vi "Request Vecto Info.vi"(8 "error in (no error)":errorcluster, 9 "Timeout mS (1000)":i32=1000, 11 "VectoService in":refnum<class "VectoInfo.lvclass">) -> (0 "error out":errorcluster, 2 "Vecto Info":T1, 3 "VectoService out":refnum<class "VectoInfo.lvclass">)   [LabVIEW 2020, in "Vecto.lvlib" / "VectoInfo.lvclass"]
uses:
  VectoInfo.lvclass
  lv-promises/Promises/Future/Future.lvclass
  lv-promises/Promises/Promise/Promise.lvclass
  VectoInfoValue/VectoInfoValue.lvclass
  Connection Type.ctl
  Vecto.lvlib
  Connection Info.ctl
  Vecto Info.ctl
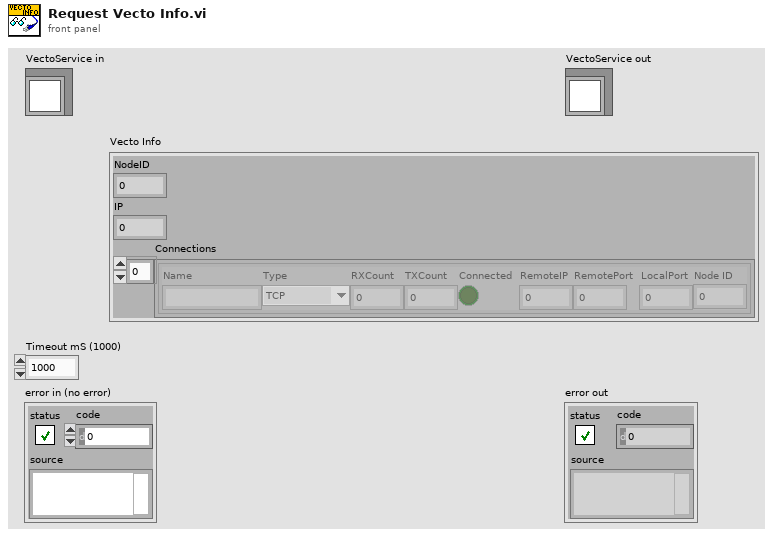
[diagram p1: front panel]
types:
  T1 = typedef "Vecto.lvlib/Vecto Info.ctl" = cluster{"NodeID":i32, "IP":u32, "Connections":T2[]}
  T2 = typedef "Vecto.lvlib/Connection Info.ctl" = cluster{"Name":string, "Type":T3, "RXCount":i32, "TXCount":i32, "Connected":bool, "RemoteIP":u32, "RemotePort":u16, "LocalPort":u16, "Node ID":u32}
  T3 = typedef "Vecto.lvlib/Connection Type.ctl" = enum16{"TCP", "Telemetry", "Discovery", "HTTP"}
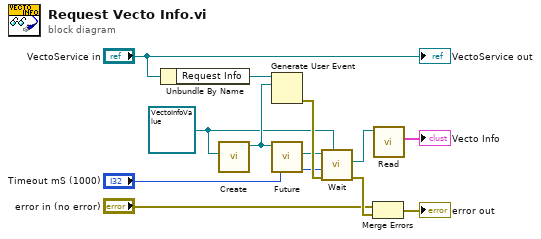
[diagram p0: block diagram]
diagram:
  w6 = refnum<class "VectoInfoValue.lvclass"> refnum ("Vecto.lvlib:VectoInfoValue.lvclass")
  n1 = Unbundle By Name("VectoService in") -> ("Request Info"=w9:refnum<user-event>)
  n2 = call "Create.vi"("Result Type"=w6) -> ("Promise"=w8:refnum<class "Promise.lvclass">)  [unwired: 9 in, 1 out]
  n3 = Generate User Event(user event=w9, event data cluster=w8) -> (error out=w12:errorcluster)  [unwired: 2 in, 1 out]
  n4 = call "Future.vi"("Promise in"=w8) -> ("Future"=w11:refnum<class "Future.lvclass">)  [unwired: 9 in, 1 out]
  n5 = call "Wait.vi"("Result Type"=w6, "error in (no error)"=w12, "Timeout mS (-1)"="Timeout mS (1000)", "Future in"=w11) -> ("error out"=w3:errorcluster, "Result"=w5:refnum<class "VectoInfoValue.lvclass">)  [unwired: 6 in]
  n6 = Merge Errors("error in (no error)", w3) -> (→"error out":errorcluster)
  n7 = call "Read.vi"("VectoInfoValue in"=w5) -> ("Vecto Info"=→"Vecto Info":T1)  [unwired: 10 in]
  "VectoService out" <- "VectoService in"
